vi "Temperature Limit.vi"(3 "상위 리미트":dbl=80.0 format="%.2f", 5 "수집할 포인트":i32=75 min=20 max=500) -> ()   [LabVIEW 2010]
doc: "이 VI는 온도 수집을 시뮬레이션하고 온도를 그래프에 그리고 온도가 한계를 초과할 때 사용자에게 알립니다."
panel:
  in  "델타 t (ms)":u32=400
  out "리미트 초과":bool
  in  "강제 종료":bool
  out "온도":cluster{"Temperature":dbl, "High Limit":dbl}(graph)
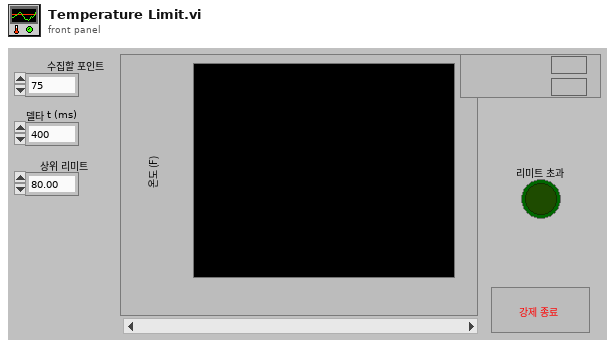
[diagram p1: front panel]
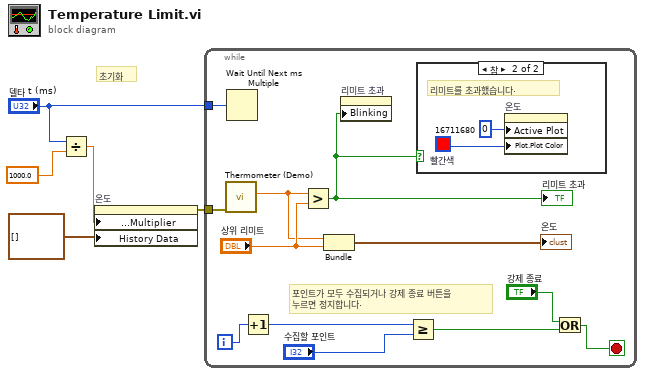
[diagram p0: block diagram]
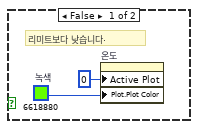
[diagram p2: hidden frame]
diagram:
  # "초기화"
  n1 = Divide(x="델타 t (ms)", y=1000.0) -> (x/y=w1:dbl)
  n2 = property on="온도" class="WFChart (엄격한)"("X Scale.Offset and Multiplier:Multiplier"=w1, "History Data"=cluster{"Temperature":dbl, "High Limit":dbl}[] []) -> (error out=w4:errorcluster)  [unwired: 2 in, 1 out]
  n3 = while {
    tunnel: "델타 t (ms)" -> [w9]
    tunnel: w4 -> [w7]
    i -> [w16]
    stop <- w10 stop-if-true
    # "포인트가 모두 수집되거나 강제 종료 버튼을 누르면 정지합니다."
    n4 = call "Thermometer (Demo).vi"("에러 입력(에러 없음)"=w7) -> ("온도"=w6:dbl)  [unwired: 9 in, 1 out]
    n5 = Wait Until Next ms Multiple(millisecond multiple=w9) -> ()  [unwired: 1 out]
    n6 = Increment(x=w16) -> (x+1=w14:i32)
    n7 = Greater?(x=w6, y="상위 리미트") -> (0:w8:bool)
    "리미트 초과" <- w8
    n8 = Bundle("온도"=w6, "상위 리미트"="상위 리미트") -> (→"온도":cluster{"온도":dbl, "상위 리미트":dbl})  [unwired: 1 in]
    n9 = property on="리미트 초과" class="Bool (엄격한)"("Blinking"=w8) -> ()  [unwired: 2 in, 2 out]
    n10 = Greater Or Equal?(x=w14, y="수집할 포인트") -> (x >= y?=w12:bool)
    n11 = case shown="참" w8 {
      frame False {
        w18 = u32 6618880  # 녹색
        # "리미트보다 낮습니다."
        n12 = property on="온도" class="WFChart (엄격한)"("Active Plot"=u32 0, "Plot.Plot Color"=w18) -> ()  [unwired: 2 in, 2 out]
      }
      frame True {
        w21 = u32 16711680  # 빨간색
        # "리미트를 초과했습니다."
        n13 = property on="온도" class="WFChart (엄격한)"("Active Plot"=u32 0, "Plot.Plot Color"=w21) -> ()  [unwired: 2 in, 2 out]
      }
    }
    n14 = Or(x="강제 종료", y=w12) -> (x .or. y?=w10:bool)
  }
